vi "placeOrders.vi"(8 "error in (no error)":errorcluster, 11 "Broker in":refnum<class "Broker.lvclass">) -> (0 "error out":errorcluster, 3 "Broker out":refnum<class "Broker.lvclass">)   [LabVIEW 2018, in "Broker.lvclass"]
uses:
  Broker.lvclass
  Broker.lvclass/Broker.ctl
  Order Class/Order.lvclass
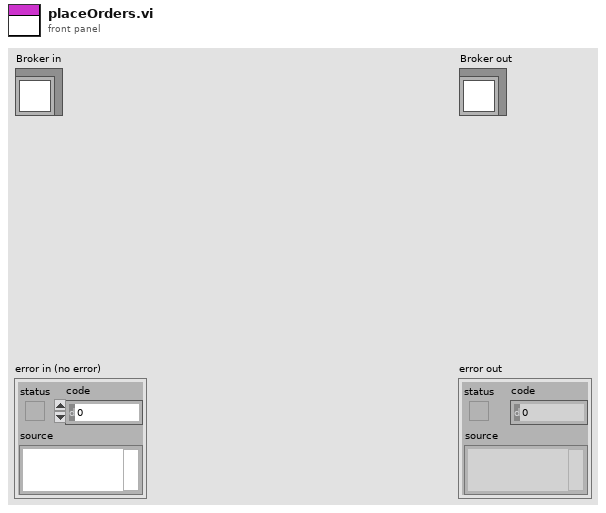
[diagram p1: front panel]
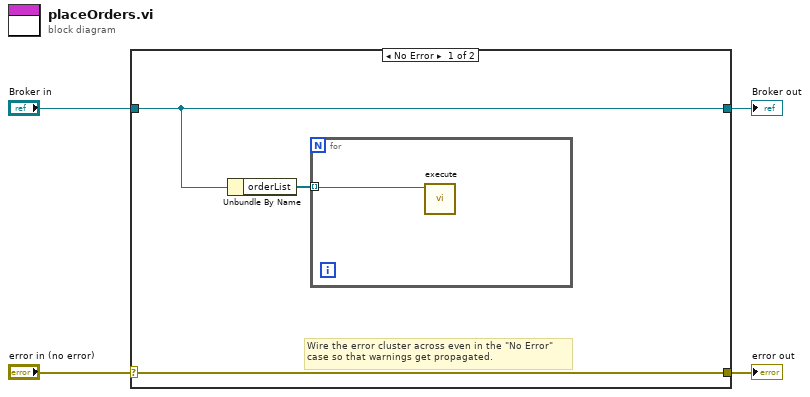
[diagram p0: block diagram]
diagram:
  n1 = case shown="No Error" "error in (no error)" {
    selector: "error in (no error)" -> [w7 w10]
    tunnel: [w7 w10] -> w3
    tunnel: [w6 w9] -> w1
    tunnel: "Broker in" -> [w6 w9]
    frame No Error {
      # "Wire the error cluster across even in the \"No Error\"\ncase so that warnings get propagated."
      n2 = Unbundle By Name(w6) -> ("orderList"=w5:refnum<class "Order.lvclass">[])
      n3 = for {
        tunnel: w5 -> [w8] mode=indexing
        n4 = call-dynamic "execute.vi"("Order in"=w8) -> ()  [unwired: 9 in, 2 out]
      }
    }
    frame Error {
    }
  }
  "error out" <- w3
  "Broker out" <- w1
